vi "VCS Get Position Compare Parameter.vi"(6 "error in (no error)":errorcluster, 9 "axis in":cluster{"keyHandle":u32, "nodeId":u16}={"keyHandle"=0, "nodeId"=1}) -> (0 "error out":errorcluster, 2 "position compare parameter":T1 {"operationalMode" items=["single position mode", "position sequence mode"]; "intervalMode" items=["negative direction to reference position", "positive direction to reference position", "positive and negative direction to reference position"]; "directionDependency" items=["negative motor direction", "positive motor direction", "both motor direction"]}, 3 "axis out":cluster{"keyHandle":u32, "nodeId":u16}={"keyHandle"=0, "nodeId"=1})   [LabVIEW 2010]
doc: "<B>VCS_GetPositionCompareParameter</B> reads all parameters for position compare."
uses:
  Resources/EposCmd.dll
  Resources/EposCmd64.dll
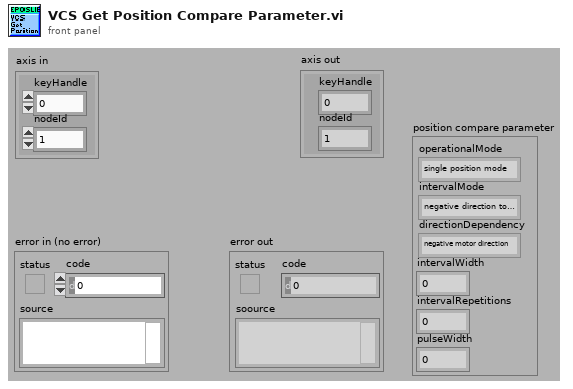
[diagram p1: front panel]
types:
  T1 = cluster{"operationalMode":u8, "intervalMode":u8, "directionDependency":u8, "intervalWidth":u16, "intervalRepetitions":u16, "pulseWidth":u16}
  T2 = cluster{"pOperationalMode":u8, "pIntervalMode":u8, "pDirectionDependency":u8, "pIntervalWidth":u16, "pIntervalRepetitions":u16, "pPulseWidth":u16}
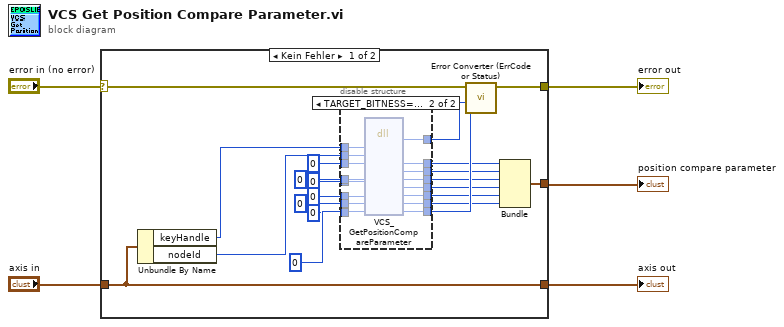
[diagram p0: block diagram]
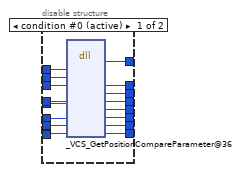
[diagram p2: hidden frame]
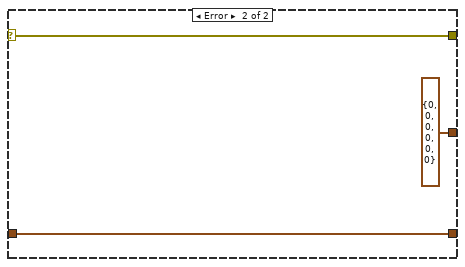
[diagram p3: hidden frame]
diagram:
  n1 = case shown="Kein Fehler" "error in (no error)" {
    selector: "error in (no error)" -> [w24 w62]
    tunnel: "axis in" -> [w26 w63]
    tunnel: [w26 w63] -> w4
    tunnel: [w25 w62] -> w3
    tunnel: [w12 T2 {"pOperationalMode"=0, "pIntervalMode"=0, "pDirectionDependency"=0, "pIntervalWidth"=0, "pIntervalRepetitions"=0, "pPulseWidth"=0}] -> w1
    frame No Error {
      n2 = Unbundle By Name(w26) -> ("keyHandle"=w20:u32, "nodeId"=w19:u16)
      n3 = disable-structure shown="TARGET_BITNESS==64" {
        disable-tunnel: u32 0 ("pErrorCode") -> [w43 w60]
        disable-tunnel: [w42 w59] -> w22
        disable-tunnel: [w41 w58] -> w21
        disable-tunnel: w20 -> [w40 w57]
        disable-tunnel: w19 -> [w39 w56]
        disable-tunnel: [w38 w55] -> w18
        disable-tunnel: [w37 w54] -> w17
        disable-tunnel: [w36 w53] -> w16
        disable-tunnel: [w35 w52] -> w15
        disable-tunnel: [w34 w51] -> w14
        disable-tunnel: [w33 w50] -> w13
        disable-tunnel: u8 0 ("pOperationalMode") -> [w32 w49]
        disable-tunnel: u8 0 ("pIntervalMode") -> [w31 w48]
        disable-tunnel: u8 0 ("pDirectionDependency") -> [w30 w47]
        disable-tunnel: u16 0 ("pIntervalWidth") -> [w29 w46]
        disable-tunnel: u16 0 ("pIntervalRepetitions") -> [w28 w45]
        disable-tunnel: u16 0 ("pPulseWidth") -> [w27 w44]
        frame condition #0 (active) {
          n4 = dll-call lib="C:/Sources/LabView/maxon EPOS/Resources/EposCmd.*" fn="_VCS_GetPositionCompareParameter@36"("KeyHandle"=w40, "NodeId"=w39, "pOperationalMode"=w32, "pIntervalMode"=w31, "pDirectionDependency"=w30, "pIntervalWidth"=w29, "pIntervalRepetitions"=w28, "pPulseWidth"=w27, "pErrorCode"=w43) -> ("Rückgabetyp"=w41:i32, "pOperationalMode"=w38:u8, "pIntervalMode"=w37:u8, "pDirectionDependency"=w36:u8, "pIntervalWidth"=w35:u16, "pIntervalRepetitions"=w34:u16, "pPulseWidth"=w33:u16, "pErrorCode"=w42:u32)  [unwired: 5 in, 2 out]
        }
        frame condition #1 {
          n5 = dll-call lib="C:/setup/Resources/EposCmd64.*" fn="VCS_GetPositionCompareParameter" ("EposCmd.dll:_VCS_GetPositionCompareParameter@36")("KeyHandle"=w57, "NodeId"=w56, "pOperationalMode"=w49, "pIntervalMode"=w48, "pDirectionDependency"=w47, "pIntervalWidth"=w46, "pIntervalRepetitions"=w45, "pPulseWidth"=w44, "pErrorCode"=w60) -> ("Rückgabetyp"=w58:i32, "pOperationalMode"=w55:u8, "pIntervalMode"=w54:u8, "pDirectionDependency"=w53:u8, "pIntervalWidth"=w52:u16, "pIntervalRepetitions"=w51:u16, "pPulseWidth"=w50:u16, "pErrorCode"=w59:u32)  [unwired: 5 in, 2 out]
        }
      }
      n6 = call "Error Converter (ErrCode or Status).vi"("error code"=w22, "return type"=w21, "error in (no error)"=w24) -> ("error out"=w25:errorcluster)  [unwired: 7 in]
      n7 = Bundle("pOperationalMode"=w18, "pIntervalMode"=w17, "pDirectionDependency"=w16, "pIntervalWidth"=w15, "pIntervalRepetitions"=w14, "pPulseWidth"=w13) -> (w12:T2)  [unwired: 1 in]
    }
    frame Error {
    }
  }
  "error out" <- w3
  "axis out" <- w4
  "position compare parameter" <- w1
